vi "Set Payload.vi"(7 "Msg":refnum<class "Msg.lvclass">, 11 "Payload":T1) -> (5 "Msg":refnum<class "Msg.lvclass">)   [LabVIEW 2020, in "_Template.lvlib" / "{{Msg}}.lvlib" / "Msg.lvclass"]
uses:
  Msg.lvclass
  Msg.lvclass/Msg.ctl
  Payload.ctl
  {{Msg}}.lvlib
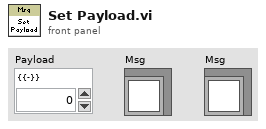
[diagram p1: front panel]
types:
  T1 = typedef "_Template.lvlib/{{Msg}}.lvlib/Payload.ctl" = cluster{"{{-}}":u8}
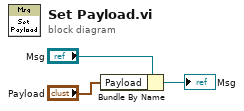
[diagram p0: block diagram]
diagram:
  n1 = Bundle By Name(cluster="Msg", "Payload"="Payload") -> (→"Msg":refnum<class "Msg.lvclass">)
